vi "Init (Auto).vi"(7 "Error Checking (Full)":T2=enum."Full", 8 "error in (no error)":errorcluster, 11 "VISA resource name":refnum<visa-resource-name>) -> (0 "error out":errorcluster, 2 "Identity":T1, 3 "Session":refnum<class "Session.lvclass">)   [LabVIEW 2020, in "CTI.lvlib" / "VisaComms.lvclass"]
uses:
  VisaComms.lvclass
  Session/Session.lvclass
  Error Reporting.ctl
  Identity.ctl
  CTI.lvlib
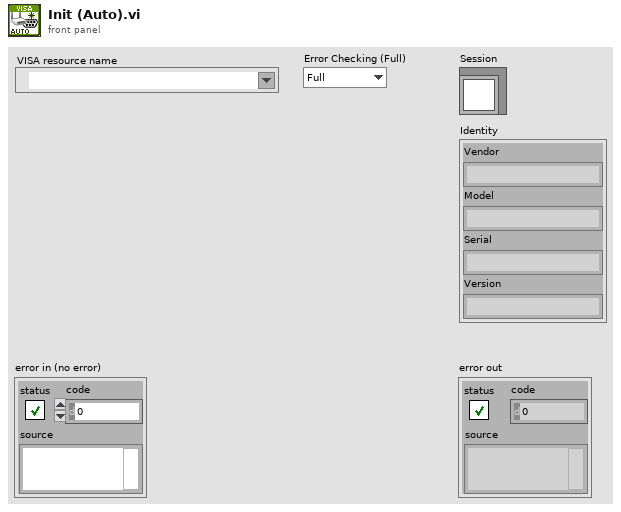
[diagram p1: front panel]
types:
  T1 = typedef "CTI.lvlib/Identity.ctl" = cluster{"Vendor":string, "Model":string, "Serial":string, "Version":string}
  T2 = typedef "CTI.lvlib/Error Reporting.ctl" = enum16{"Minimal", "Moderate", "Full"}
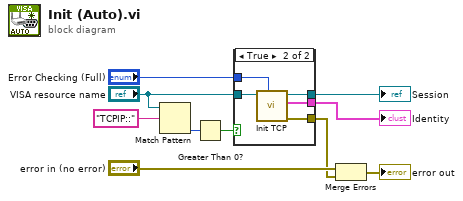
[diagram p0: block diagram]
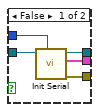
[diagram p2: hidden frame]
diagram:
  n1 = Match Pattern(string="VISA resource name", regular expression="TCPIP::") -> (offset past match=w5:i32)  [unwired: 1 in, 3 out]
  n2 = Greater Than 0?(x=w5) -> (x > 0?=w4:bool)
  n3 = case shown="True" w4 {
    tunnel: [w13 w18] -> w2
    tunnel: [w14 w19] -> w3
    tunnel: "Error Checking (Full)" -> [w12 w17]
    tunnel: "VISA resource name" -> [w15 w20]
    tunnel: [w11 w16] -> w1
    frame False {
      n4 = call "Init Serial.vi"("Error Checking (Full)"=w12, "VISA resource name in"=w15) -> ("error out"=w13:errorcluster, "Identity"=w11:T1, "Session"=w14:refnum<class "Session.lvclass">)  [unwired: 7 in]
    }
    frame True {
      n5 = call "Init TCP.vi"("Error Checking (Full)"=w17, "VISA resource name"=w20) -> ("error out"=w18:errorcluster, "Identity"=w16:T1, "Session"=w19:refnum<class "Session.lvclass">)  [unwired: 7 in]
    }
  }
  "Session" <- w3
  "Identity" <- w1
  n6 = Merge Errors("error in (no error)", w2) -> (→"error out":errorcluster)
